vi "Part 1.vi"(11 "Input":string) -> (3 "Output":i64)   [LabVIEW 2021]
uses:
  639bc2a2-0f5b-4fb3-bd8c-bb8634648e7f.vi
  55c09d35-bafa-4441-b3a3-390b9bd4dfee.vi
  <userlib>/_OpenG.lib/string/string.llb/Convert EOLs (String)__ogtk.vi
panel:
  out "Array 3":cluster{"array":i32[]}[](array[cluster])
  out "Array 2":i32[](array[numeric])
  in  "Input 2":string
  out "Array":cluster{"array":i32[]}[](array[cluster])
  out "max z":i32
  out "max y":i32
  out "max x":i32
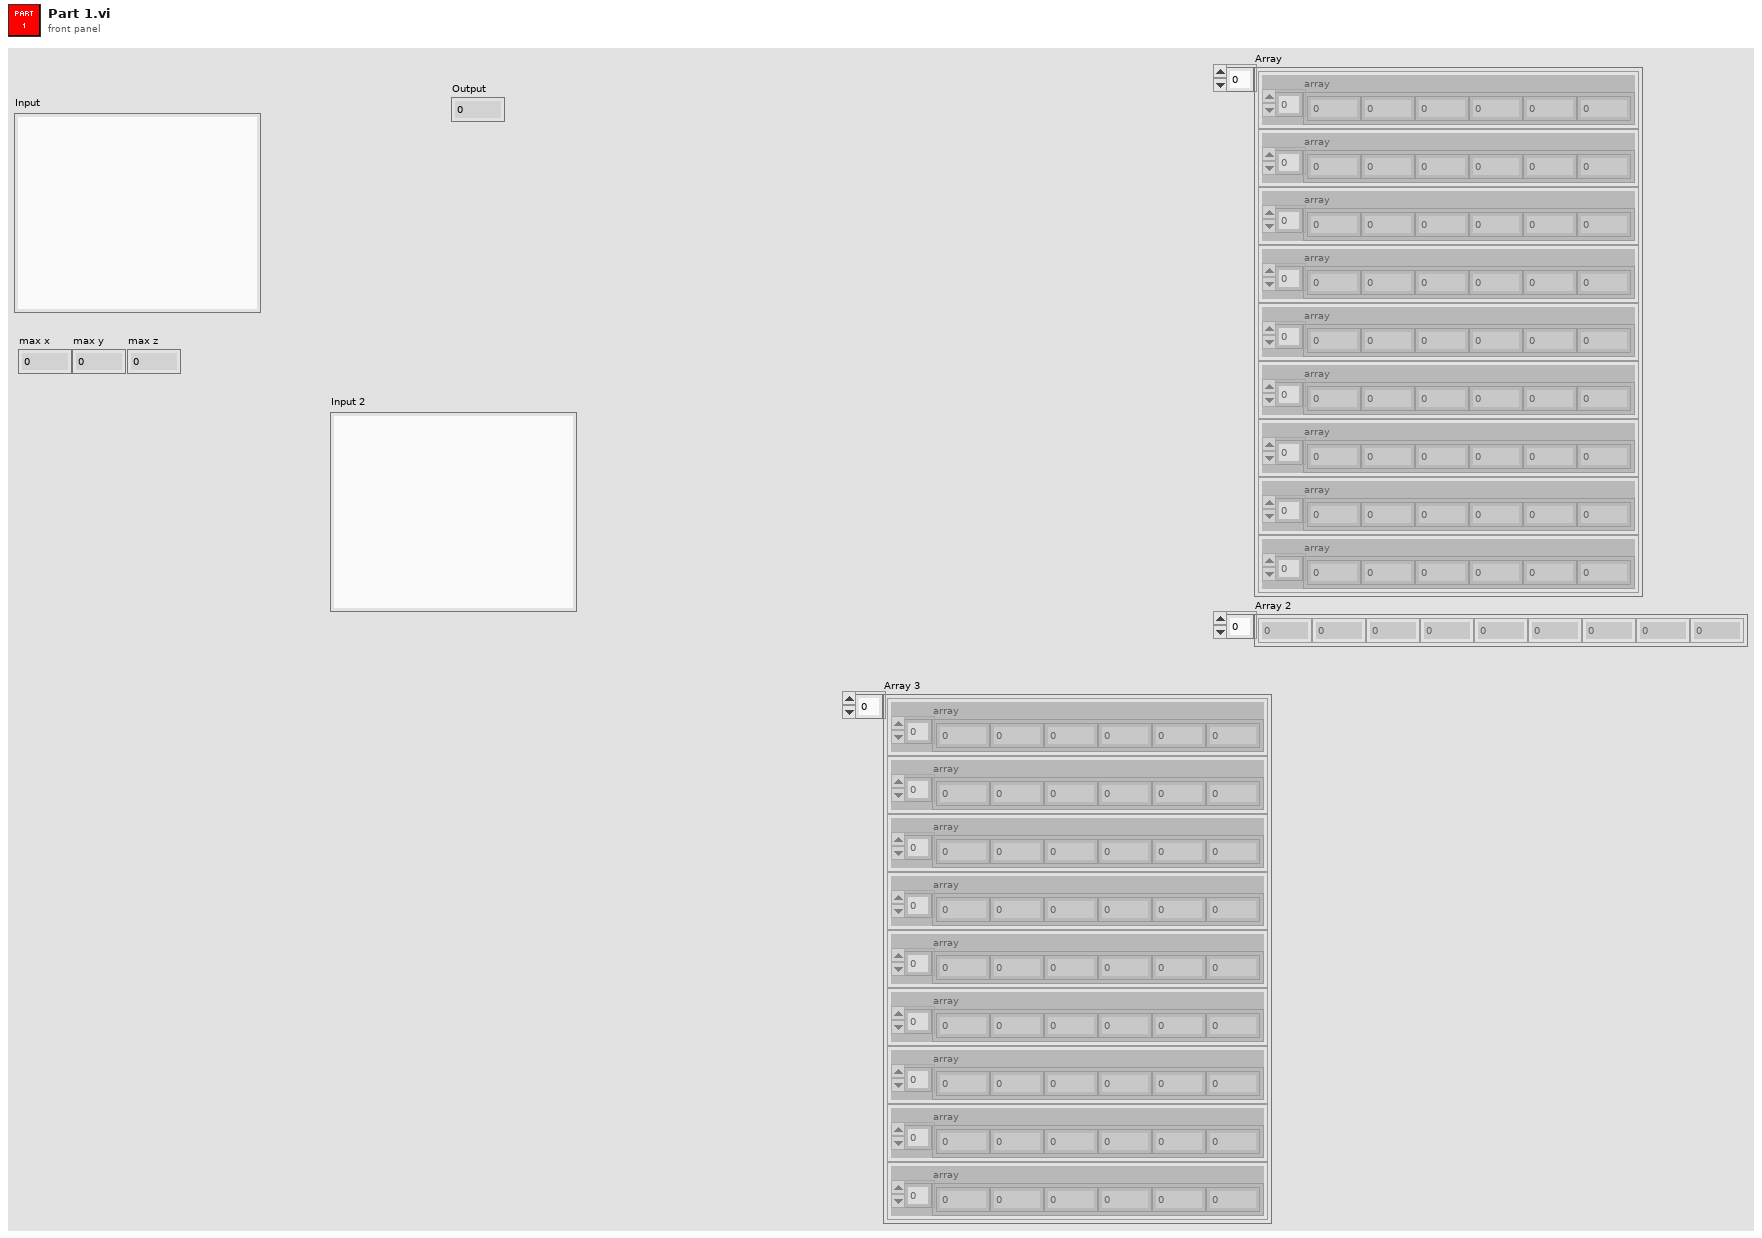
[diagram p1: front panel]
types:
  T1 = cluster{"array with duplicates removed":cluster{i32, i32, i32}[]}
  T2 = cluster{"array with duplicates removed":cluster{i32, i32, i32}[]}[]
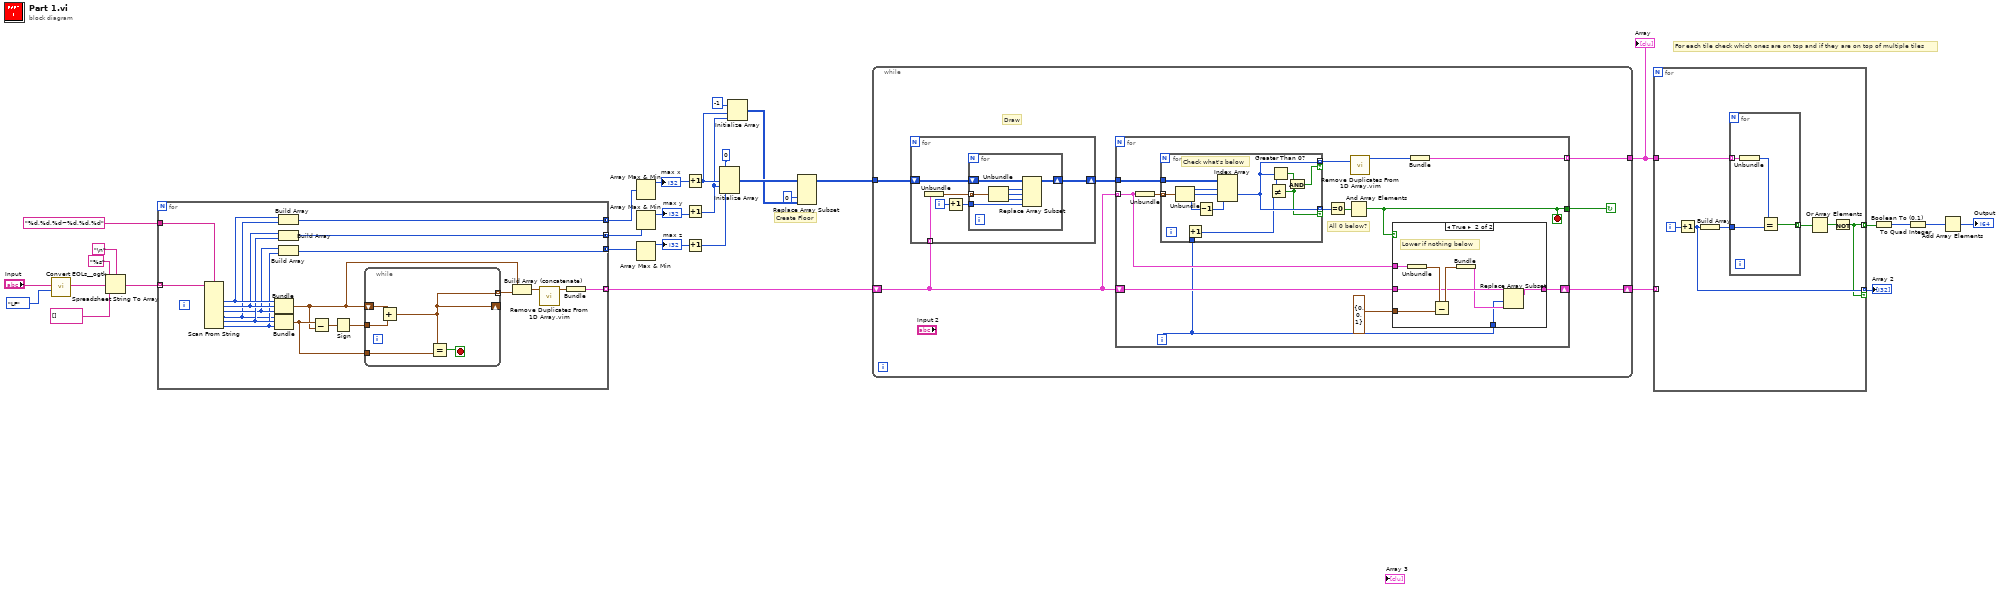
[diagram p0: block diagram]
diagram:
  # "Create Floor"
  # "For each tile check which ones are on top and if they are on top of multiple tiles"
  n1 = call-poly <userlib>:"Convert EOLs__ogtk.vi"("Convert to:"=enum16{"CR", "LF", "CRLF"}."LF", "String in"="Input") -> ("String out"=w27:string)  [unwired: 9 in]
  n2 = Spreadsheet String To Array(delimiter (Tab)="\n", format string="%s", spreadsheet string=w27, array type (2D Dbl)=string[] []) -> (array=w25:string[])
  n3 = for {
    tunnel: w25 -> [w50] mode=indexing
    tunnel: "%d,%d,%d~%d,%d,%d" ("delimiter (Tab)") -> [w49]
    tunnel: [w43] -> w15 mode=indexing
    tunnel: [w35] -> w21 mode=concatenating
    tunnel: [w34] -> w22 mode=concatenating
    tunnel: [w33] -> w23 mode=concatenating
    n4 = Scan From String(format string=w49, input string=w50) -> (output 1=w40:i32, output 2=w39:i32, output 3=w37:i32, output 4=w32:i32, output 5=w38:i32, output 6=w36:i32)  [unwired: 8 in, 3 out]
    n5 = Bundle(w40, w39, w37) -> (w44:cluster{i32, i32, i32})  [unwired: 1 in]
    n6 = Bundle(w32, w38, w36) -> (w46:cluster{i32, i32, i32})  [unwired: 1 in]
    n7 = Build Array(w40, w32) -> (w35:i32[])
    n8 = Build Array(w39, w38) -> (w34:i32[])
    n9 = Build Array(w37, w36) -> (w33:i32[])
    n10 = Subtract(x=w46, y=w44) -> (x-y=w48:cluster{i32, i32, i32})
    n11 = Sign(1:w48) -> (0:w47:cluster{i32, i32, i32})
    n12 = while {
      tunnel: w47 -> [w53]
      shift-right: [w51] -> _
      shift-left: w44 -> [w52]
      tunnel: w46 -> [w55]
      tunnel: [w51] -> w45 mode=indexing
      stop <- w54 stop-if-true
      n13 = Add(x=w52, y=w53) -> (x+y=w51:cluster{i32, i32, i32})
      n14 = Equal?(x=w51, y=w55) -> (x = y?=w54:bool)
    }
    n15 = Build Array (concatenate)(w44, w45) -> (w42:cluster{i32, i32, i32}[])
    n16 = call "Remove Duplicates From 1D Array.vim"("array"=w42) -> ("array with duplicates removed"=w41:cluster{i32, i32, i32}[])  [unwired: 10 in]
    n17 = Bundle("array with duplicates removed"=w41) -> (w43:T1)  [unwired: 1 in]
  }
  n18 = Array Max & Min(array=w21) -> (max value=w20:i32)  [unwired: 3 out]
  "max x" <- w20
  n19 = Array Max & Min(array=w22) -> (max value=w19:i32)  [unwired: 3 out]
  "max y" <- w19
  n20 = Array Max & Min(array=w23) -> (max value=w18:i32)  [unwired: 3 out]
  "max z" <- w18
  n21 = Increment(x=w20) -> (x+1=w12:i32)
  n22 = Increment(x=w19) -> (x+1=w11:i32)
  n23 = Increment(x=w18) -> (x+1=w17:i32)
  n24 = Initialize Array(0, w12, w11, w17) -> (w16:i32[][][])
  n25 = Initialize Array(-1, w12, w11) -> (w8:i32[][])
  n26 = Replace Array Subset(array=w16, new element=w8, index (dim 2)=0 ("disabled index (col)")) -> (w14:i32[][][])  [unwired: 2 in]
  n27 = while {
    shift-right: [w59] -> w6
    shift-left: w15 -> [w56]
    tunnel: [w58] -> w7
    tunnel: w14 -> [w61]
    stop <- w57 continue-if-true
    # "Draw"
    n28 = for {
      shift-right: [w100] -> w60
      shift-left: w61 -> [w101]
      tunnel: w56 -> [w97] mode=indexing
      i -> [w98]
      n29 = Unbundle(w97) -> ("array with duplicates removed"=w99:cluster{i32, i32, i32}[])
      n30 = Increment(x=w98) -> (x+1=w96:i32)
      n31 = for {
        shift-right: [w103] -> w100
        shift-left: w101 -> [w107]
        tunnel: w99 -> [w108] mode=indexing
        tunnel: w96 -> [w102]
        n32 = Unbundle(w108) -> (w106:i32, w105:i32, w104:i32)
        n33 = Replace Array Subset(array=w107, new element=w102, index (dim 0)=w106, index (dim 1)=w105, index (dim 2)=w104) -> (w103:i32[][][])
      }
    }
    n34 = for {
      tunnel: [w64] -> w57
      tunnel: [w68] -> w58 mode=indexing
      shift-right: [w70] -> w59
      shift-left: w56 -> [w71]
      tunnel: w56 -> [w63] mode=indexing
      tunnel: w60 -> [w74]
      i -> [w62]
      stop <- w64 stop-if-true
      # "All 0 below?"
      n35 = Unbundle(w63) -> ("array with duplicates removed"=w73:cluster{i32, i32, i32}[])
      n36 = for {
        tunnel: w73 -> [w95] mode=indexing
        tunnel: [w89] -> w69 mode=indexing if=w86
        tunnel: [w89] -> w66 mode=indexing if=w87
        tunnel: w74 -> [w92]
        tunnel: w62 -> [w84]
        # "Check what's below"
        n37 = Unbundle(w95) -> (w94:i32, w93:i32, w91:i32)
        n38 = Increment(x=w84) -> (x+1=w85:i32)
        n39 = Decrement(x=w91) -> (x-1=w90:i32)
        n40 = Index Array(array=w92, index (dim 0)=w94, index (dim 1)=w93, index (dim 2)=w90) -> (element=w89:i32)
        n41 = Not Equal?(x=w89, y=w85) -> (x != y?=w86:bool)
        n42 = Greater Than 0?(x=w89) -> (x > 0?=w88:bool)
        n43 = And(x=w88, y=w86) -> (x .and. y?=w87:bool)
      }
      n44 = Equal To 0?(x=w69) -> (x = 0?=w72:bool[])
      n45 = And Array Elements(Boolean array=w72) -> (logical AND=w64:bool)
      n46 = call "Remove Duplicates From 1D Array.vim"("array"=w66) -> ("array with duplicates removed"=w65:i32[])  [unwired: 10 in]
      n47 = case shown="True" w64 {
        tunnel: w71 -> [w75 w79]
        tunnel: [w75 w77] -> w70
        tunnel: cluster{i32, i32, i32} {0, 0, 1} -> [_ w82]
        tunnel: w63 -> [_ w80]
        tunnel: w62 -> [_ w76]
        frame False {
        }
        frame True {
          # "Lower if nothing below"
          n48 = Unbundle(w80) -> ("array with duplicates removed"=w83:cluster{i32, i32, i32}[])
          n49 = Subtract(x=w83, y=w82) -> (x-y=w81:cluster{i32, i32, i32}[])
          n50 = Bundle(w81) -> (w78:cluster{cluster{i32, i32, i32}[]})  [unwired: 1 in]
          n51 = Replace Array Subset(array=w79, new element=w78, index=w76) -> (w77:T2)
        }
      }
      n52 = Bundle("array with duplicates removed"=w65) -> (w68:cluster{"array with duplicates removed":i32[]})  [unwired: 1 in]
    }
  }
  "Array" <- w7
  n53 = for {
    tunnel: w7 -> [w115]
    tunnel: w6 -> [_] mode=indexing
    tunnel: [w109] -> w5 mode=indexing
    tunnel: [w110] -> w1 mode=indexing if=w109
    i -> [w114]
    n54 = Increment(x=w114) -> (x+1=w110:i32)
    n55 = Build Array(w110) -> (w113:i32[])
    n56 = for {
      tunnel: w115 -> [w119] mode=indexing
      tunnel: w113 -> [w118]
      tunnel: [w116] -> w112 mode=indexing
      n57 = Unbundle(w119) -> ("array with duplicates removed"=w117:i32[])
      n58 = Equal?(x=w117, y=w118) -> (x = y?=w116:bool)
    }
    n59 = Or Array Elements(Boolean array=w112) -> (logical OR=w111:bool)
    n60 = Not(x=w111) -> (.not. x?=w109:bool)
  }
  "Array 2" <- w1
  n61 = Boolean To (0,1)(Boolean=w5) -> (0, 1=w4:i16[])
  n62 = To Quad Integer(1:w4) -> (0:w2:i64[])
  n63 = Add Array Elements(numeric array=w2) -> (sum=→"Output":i64)
